vi "Read EXT.vi"(8 "error in (no error)":errorcluster, 9 "Default If Not Found":ext, 10 "Name":string, 11 "IConfiguration in":refnum<class "IConfiguration.lvclass">) -> (0 "error out":errorcluster, 1 "Not Found?":bool, 2 "Value":ext, 3 "IConfiguration out":refnum<class "IConfiguration.lvclass">)   [LabVIEW 2017, in "Configuration.lvlib" / "IConfiguration.lvclass"]
uses:
  IConfiguration.lvclass
  <vilib>/Utility/Data Type/Type Definitions/Data Type.ctl
  <vilib>/Utility/Data Type/NI_Data Type.lvlib
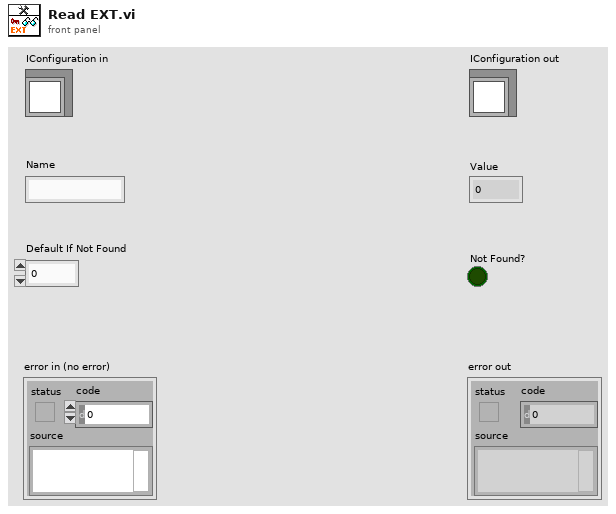
[diagram p1: front panel]
types:
  T1 = typedef "NI_Data Type.lvlib/Data Type.ctl" = enum8{"Invalid Type", "Void", "I8", "I16", "I32", "I64", "U8", "U16", "U32", "U64", "Single Float", "Double Float", "Extended Float", "Single Complex", "Double Complex", "Extended Complex", "Enum U8", "Enum U16", "Enum U32", "Enum U64", "Single Float With Unit", "Double Float With Unit", "Extended Float With Unit", "Single Complex with Unit", "Double Complex with Unit", "Extended Complex with Unit", "Boolean", "String", "Path", "Picture", "Tag", "Array", "Cluster", "Variant", "LV Variant", "Waveform", "Timestamp", "Digital Waveform", "Digital Data", "ExpressData", "Refnum", "External Data", "VI", "Poly VI", "LabVIEW Class Instance", "Fixed Point"}
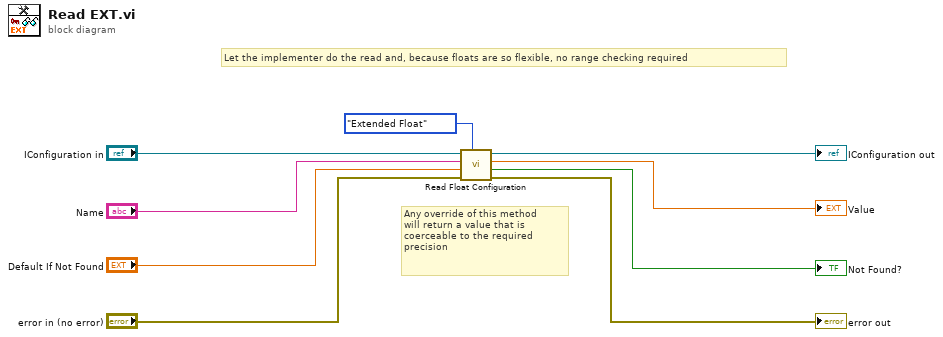
[diagram p0: block diagram]
diagram:
  # "Any override of this method\nwill return a value that is\ncoerceable to the required\nprecision"
  # "Let the implementer do the read and, because floats are so flexible, no range checking required"
  n1 = call-dynamic "Read Float Configuration.vi"("Type"=Data_Type."Extended Float", "error in (no error)"="error in (no error)", "Default If Not Found"="Default If Not Found", "Name"="Name", "IConfiguration in"="IConfiguration in") -> ("error out"=→"error out":errorcluster, "Not Found?"=→"Not Found?":bool, "Value"=→"Value":ext, "IConfiguration out"=→"IConfiguration out":refnum<class "IConfiguration.lvclass">)  [unwired: 3 in]
